vi "WPI_CameraSend Images To PC LoopCustom2.vi"(8 "error in (no error)":errorcluster, 11 "CameraDevRef":T1) -> ()   [LabVIEW 2015]
doc: "This VI is used to send images to the dashboard using the second enet port on the 8 slot controller. This is provided for compatibility, but is higher overhead than using the Camera MJPG approach.\n\nThis software is licensed. Open the labview\\readme\\WPI Robotics Library Open Source License.txt file for more information."
uses:
  <vilib>/Rock Robotics/WPI/Camera/WPI_CameraDevRef.ctl
  <vilib>/Rock Robotics/SystemInterfaces/NetworkCommunication/NetComm_UsageReport_ResourceType.ctl
  Robot Global Data.vi
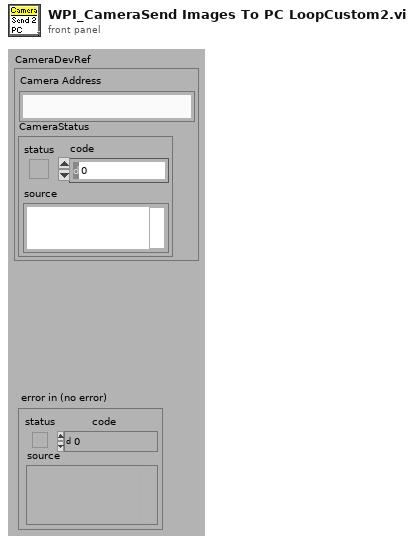
[diagram p1: front panel]
types:
  T1 = typedef "WPI_CameraDevRef.ctl" = cluster{"Camera Address":string, "CameraStatus":errorcluster}
  T2 = cluster{"fps":i32, "compression":i32, "compression 2":i32}
  T3 = typedef "NetComm_UsageReport_ResourceType.ctl" = enum8{"Controller", "Module", "Language", "CANPlugin", "Accelerometer", "ADXL345", "AnalogChannel", "AnalogTrigger", "AnalogTriggerOutput", "CANJaguar", "Compressor", "Counter", "Dashboard", "DigitalInput", "DigitalOutput", "DriverStationCIO", "DriverStationEIO", "DriverStationLCD", "Encoder", "GearTooth", "Gyro", "I2C", "Framework", "Jaguar", "Joystick", "Kinect", "KinectStick", "PIDController", "Preferences", "PWM", "Relay", "RobotDrive", "SerialPort", "Servo", "Solenoid", "SPI", "Task", "Ultrasonic", "Victor", "Button", "Command", "AxisCamera", "PCVideoServer", "SmartDashboard", "Talon", "HiTechnicColorSensor", "HiTechnicAccel", "HiTechnicCompass", "SRF08", "AnalogOutput", "Victor SP", "Talon SRX", "CAN Talon SRX", "ADXL362 Accel", "ADXRS450 Gyro", "Rev SPARK", "Mindsensors SD540", "Digital Filter"}
  T4 = enum16{"Update Mode", "Get Image", "Get Image Data"}
  T5 = typedef "Image Type" = u32
  T6 = typedef "IMAQ Image.ctl" = refnum<image>
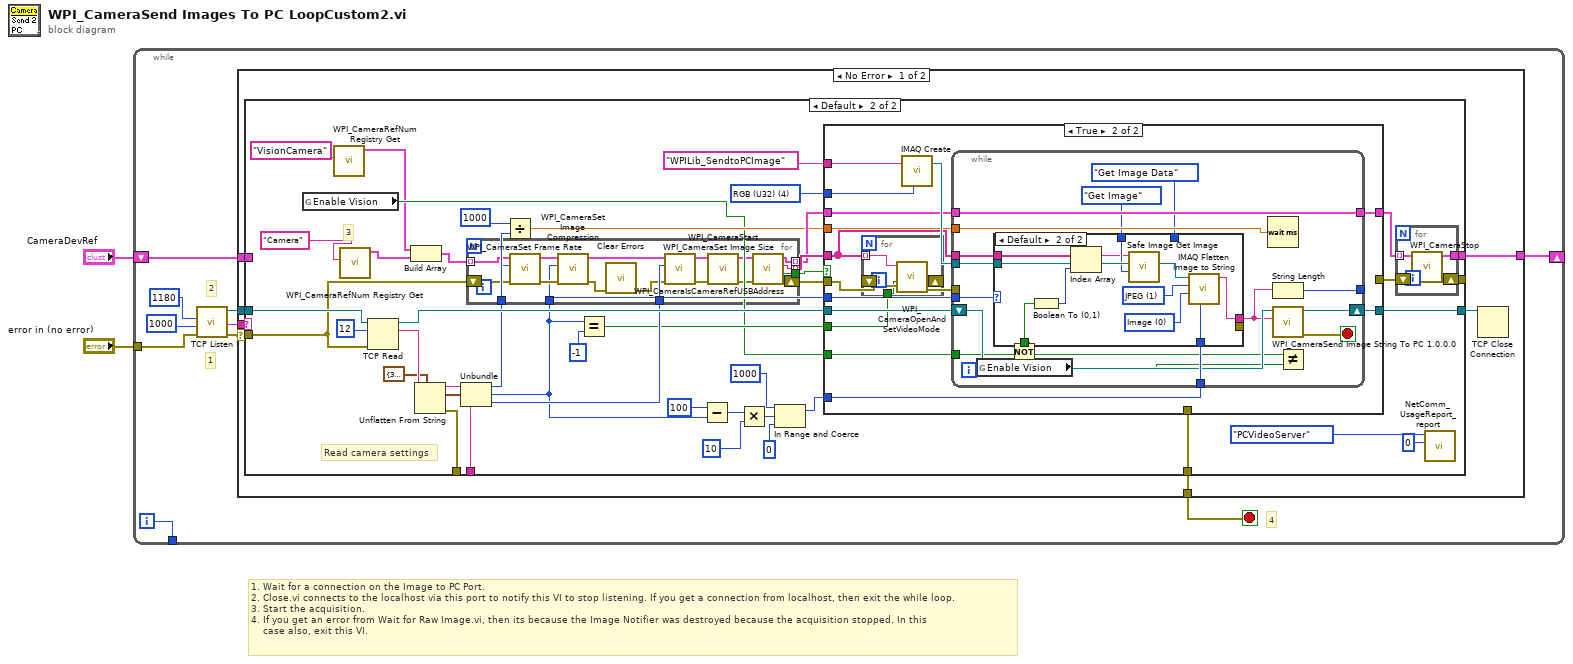
[diagram p0: block diagram]
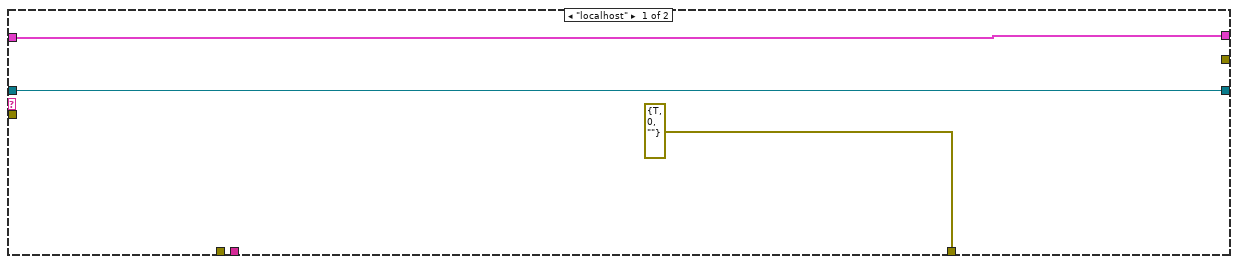
[diagram p2: hidden frame]
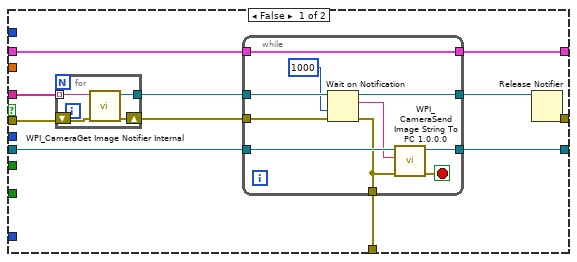
[diagram p3: hidden frame]
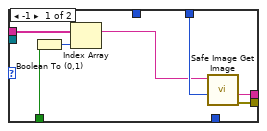
[diagram p4: hidden frame]
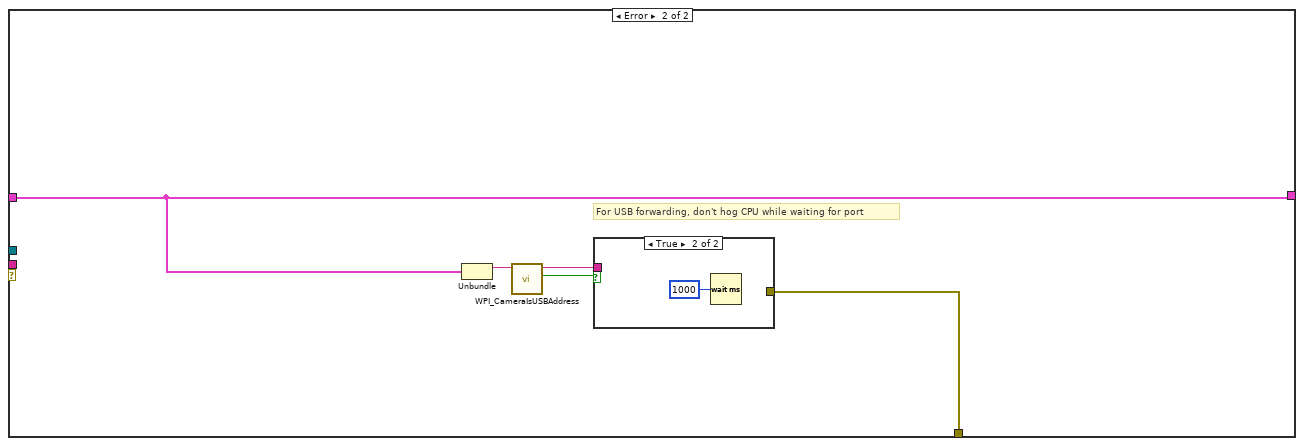
[diagram p5: hidden frame]
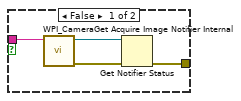
[diagram p6: hidden frame]
diagram:
  # "1. Wait for a connection on the Image to PC Port.\n2. Close.vi connects to the localhost via this port to notify this VI to stop listening. If you get a connection from localhost, then exit the while loop.\n3. Start the acquisition.\n4. If you get an error from Wait for Raw Image.vi, then its because the Image Notifier was destroyed because the acquisition stopped. In this\n    case also, exit this VI."
  n1 = while {
    tunnel: "error in (no error)" -> [w9]
    shift-right: [w12] -> _
    shift-left: "CameraDevRef" -> [w10]
    tunnel: [w3] -> _
    i -> [w3]
    stop <- w7 stop-if-true
    # "4"
    # "1"
    # "2"
    n2 = call <vilib>:"TCP Listen.vi"("error in (no error)"=w9, "timeout ms (wait forever: -1)"=u16 1000 ("port"), "port"=u16 1180) -> ("error out"=w5:errorcluster, "remote address"=w11:string, "connection ID"=w8:refnum<k5>)  [unwired: 1 in, 5 out]
    n3 = case shown="No Error" w5 {
      selector: w5 -> [w13 _]
      tunnel: [w19 w169] -> w12
      tunnel: w11 -> [w18 _]
      tunnel: w10 -> [w17 w169]
      tunnel: w8 -> [w16 _]
      tunnel: [w15 w170] -> w7
      frame No Error {
        n4 = case shown="Default" w18 {
          tunnel: [w22 w63] -> w19
          tunnel: w17 -> [w22 _]
          tunnel: w13 -> [_ w48]
          tunnel: w16 -> [w20 w52]
          tunnel: [errorcluster {"status"=TRUE, "code"=0, "source"=""} ("error out 2") w65] -> w15
          tunnel: [w20 w64] -> w14
          tunnel: [_ w62] -> _
          tunnel: [_ w31] -> _
          tunnel: [_ w30] -> _
          frame "localhost" {
          }
          frame Default {
            w57 = T5 4 items=["Grayscale (U8)", "Grayscale (I16)", "Grayscale (SGL)", "Complex (CSG)", "RGB (U32)", "HSL (U32)", "RGB (U64)", "Grayscale (U16)"] ("Image Type")
            # "Read camera settings"
            # "3"
            n5 = global read "Robot Global Data.vi" "Enable Vision"() -> (w29:bool)
            n6 = call <vilib>:"WPI_CameraRefNum Registry Get.vi"("refnum name"="VisionCamera") -> ("CameraDevRef"=w27:T1)  [unwired: 9 in, 1 out]
            n7 = call <vilib>:"WPI_CameraRefNum Registry Get.vi"("refnum name"="Camera") -> ("CameraDevRef"=w26:T1)  [unwired: 9 in, 1 out]
            n8 = TCP Read(connection ID=w52, bytes to read=12, error in (no error)=w48) -> (connection ID out=w51:refnum<k5>, data out=w49:string)  [unwired: 2 in, 1 out]
            n9 = Build Array(w27, w26) -> (w28:T1[])
            n10 = Unflatten From String(type=T2 {"fps"=30, "compression"=32, "compression 2"=32} ("Camera Settings"), binary string=w49) -> (rest of the binary string=w30:string, value=w47:T2, error out=w31:errorcluster)  [unwired: 3 in]
            n11 = Unbundle(w47) -> ("fps"=w44:i32, "compression"=w33:i32, "compression 2"=w46:i32)
            n12 = for {
              tunnel: [w87] -> w56 mode=indexing
              tunnel: [w86] -> w55
              tunnel: w46 -> [w76]
              tunnel: w44 -> [w75]
              tunnel: w33 -> [w74]
              shift-right: [w84] -> w54
              shift-left: w48 -> [w79]
              tunnel: w28 -> [w71] mode=indexing
              tunnel: [w70] -> w53 mode=indexing
              n13 = call <vilib>:"WPI_CameraSet Frame Rate.vi"("error in (no error)"=w79, "Frame Rate (fps)"=w75, "CameraDevRef"=w71) -> ("error out"=w78:errorcluster, "CameraDevRef Out"=w82:T1)  [unwired: 7 in]
              n14 = call <vilib>:"WPI_CameraSet Image Compression.vi"("error in (no error)"=w78, "Compression"=w74, "CameraDevRef"=w82) -> ("error out"=w73:errorcluster, "CameraDevRef Out"=w81:T1)  [unwired: 7 in]
              n15 = call <vilib>:"Clear Errors.vi"("error in (no error)"=w73) -> ("error out"=w72:errorcluster)  [unwired: 5 in, 1 out]
              n16 = call <vilib>:"WPI_CameraSet Image Size.vi"("error in (no error)"=w72, "Image Size"=w76, "CameraDevRef"=w81) -> ("error out"=w77:errorcluster, "CameraDevRef Out"=w80:T1)  [unwired: 7 in]
              n17 = call <vilib>:"WPI_CameraStart.vi"("error in (no error)"=w77, "CameraDevRef"=w80) -> ("error out"=w85:errorcluster, "CameraDevRef"=w83:T1)  [unwired: 8 out]
              n18 = call <vilib>:"WPI_CameraIsCameraRefUSBAddress.vi"("error in (no error)"=w85, "CameraDevRef"=w83) -> ("error out"=w84:errorcluster, "USB?"=w86:bool, "Camera Address Out"=w87:string, "CameraDevRef out"=w70:T1)  [unwired: 6 in]
            }
            n19 = Divide(x=u16 1000 ("port"), y=w44) -> (x/y=w43:dbl)
            n20 = Equal?(x=w33, y=-1) -> (x = y?=w32:bool)
            n21 = Subtract(x=100, y=w33) -> (x-y=w38:i32)
            n22 = Multiply(x=w38, y=10) -> (x*y=w40:i32)
            n23 = In Range and Coerce(upper limit=1000, x=w40, lower limit=0) -> (coerced(x)=w36:i32)  [unwired: 1 out]
            n24 = case shown="True" w55 {
              tunnel: w51 -> [w98 w127]
              tunnel: [w97 _] -> w65
              tunnel: [w96 w126] -> w64
              tunnel: w54 -> [w95 w117]
              tunnel: w56 -> [w93 w116]
              tunnel: [w92 w121] -> w25
              tunnel: w53 -> [w91 w122]
              tunnel: [w89 _] -> w61
              tunnel: "WPILib_SendtoPCImage" -> [_ w124]
              tunnel: w57 -> [_ w123]
              tunnel: w36 -> [_ w120]
              tunnel: w43 -> [_ w119]
              tunnel: w33 -> [_ w118]
              tunnel: w32 -> [_ w114]
              tunnel: w29 -> [_ w113]
              frame False {
                n25 = for {
                  tunnel: w93 -> [w100] mode=indexing
                  tunnel: [w99] -> w90
                  shift-right: [w101] -> w94
                  shift-left: w95 -> [w102]
                  n26 = call <vilib>:"WPI_CameraGet Image Notifier Internal.vi"("error in (no error)"=w102, "Camera Address"=w100) -> ("error out"=w101:errorcluster, "Image Notifier"=w99:refnum<notifier>)  [unwired: 8 out]
                }
                n27 = while {
                  tunnel: w94 -> [w108]
                  tunnel: w98 -> [w112]
                  tunnel: [w105] -> w97
                  tunnel: [w110] -> w96
                  tunnel: [w109] -> w92
                  tunnel: w91 -> [w109]
                  tunnel: w90 -> [w107]
                  tunnel: [w103] -> w88
                  stop <- w111 stop-if-true
                  n28 = Wait on Notification(notifier=w107, timeout in ms (-1)=1000 ("Timeout in ms (-1)"), error in (no error)=w108) -> (notifier out=w103:refnum<notifier>, notification=w106:string, error out=w105:errorcluster)  [unwired: 2 out]
                  n29 = call <vilib>:"WPI_CameraSend Image String To PC 1.0.0.0.vi"("error in (no error)"=w105, "String"=w106, "TCP Connection ID"=w112) -> ("error out"=w111:errorcluster, "TCP Connection ID out"=w110:refnum<k5>)  [unwired: 7 out]
                }
                n30 = Release Notifier(notifier=w88) -> (error out=w89:errorcluster)  [unwired: 1 in, 3 out]
              }
              frame True {
                n31 = for {
                  tunnel: w116 -> [w130] mode=indexing
                  tunnel: w114 -> [w128]
                  shift-right: [w129] -> w115
                  shift-left: w117 -> [w131]
                  n32 = call <vilib>:"WPI_CameraOpenAndSetVideoMode.vi"("error in (no error)"=w131, "USB JPEG"=w128, "Camera Address Out"=w130) -> ("error out"=w129:errorcluster)  [unwired: 8 in]
                }
                n33 = call "IMAQ Create"("Image Name"=w124, "Image Type"=w123) -> ("New Image"=w125:T6)  [unwired: 3 in, 1 out]
                n34 = while {
                  tunnel: w116 -> [w146]
                  shift-right: [w147] -> w126
                  shift-left: w127 -> [w141]
                  tunnel: w125 -> [w145]
                  tunnel: [w144] -> w121
                  tunnel: w122 -> [w144]
                  tunnel: w120 -> [w143]
                  tunnel: w119 -> [w142]
                  tunnel: [w139] -> _
                  tunnel: w118 -> [w138]
                  tunnel: w115 -> [_]
                  tunnel: w113 -> [w135]
                  stop <- w134 stop-if-true
                  n35 = global read "Robot Global Data.vi" "Enable Vision"() -> (w133:bool)
                  n36 = Not(x=w133) -> (.not. x?=w132:bool)
                  n37 = case shown="Default" w138 {
                    tunnel: [w153 w165] -> w140
                    tunnel: w146 -> [w154 w161]
                    tunnel: w145 -> [_ w160]
                    tunnel: w143 -> [_ w162]
                    tunnel: [w152 _] -> _
                    tunnel: T4."Get Image Data" ("Operation") -> [w151 _]
                    tunnel: T4."Get Image" ("Operation") -> [_ w158]
                    tunnel: w132 -> [w149 w156]
                    frame -1 {
                      n38 = Boolean To (0,1)(Boolean=w149) -> (0, 1=w148:i16)
                      n39 = Index Array(array=w154, index=w148) -> (element=w150:string)
                      n40 = call <vilib>:"Safe Image Get Image.vi"("Operation"=w151, "Session In"=w150) -> ("error out"=w152:errorcluster, "Image Data String"=w153:string)  [unwired: 6 in, 2 out]
                    }
                    frame Default {
                      w163 = 0 items=["Image", "Image and Vision Info", "Reference to Image"] ("Type of Flatten (Image and Vision Info)")
                      w164 = 1 items=["None", "JPEG", "PACKED BINARY"] ("Compression (None)")
                      n41 = Boolean To (0,1)(Boolean=w156) -> (0, 1=w155:i16)
                      n42 = Index Array(array=w161, index=w155) -> (element=w157:string)
                      n43 = call <vilib>:"Safe Image Get Image.vi"("Operation"=w158, "Image In"=w160, "Session In"=w157) -> ("Image Out"=w159:T6)  [unwired: 5 in, 3 out]
                      n44 = call "IMAQ Flatten Image to String"("Quality (750)"=w162, "Type of Flatten (Image and Vision Info)"=w163, "Compression (None)"=w164, "Image"=w159) -> ("Data String"=w165:string)  [unwired: 6 in, 1 out]
                    }
                  }
                  n45 = Wait (ms)(milliseconds to wait=w142) -> ()  [unwired: 1 out]
                  n46 = String Length(string=w140) -> (length=w139:i32)
                  n47 = call <vilib>:"WPI_CameraSend Image String To PC 1.0.0.0.vi"("String"=w140, "TCP Connection ID"=w141) -> ("error out"=w134:errorcluster, "TCP Connection ID out"=w147:refnum<k5>)  [unwired: 1 in, 7 out]
                  n48 = Not Equal?(x=w135, y=w133) -> ()  [unwired: 1 out]
                }
              }
            }
            n49 = for {
              tunnel: [w69] -> w63
              tunnel: w25 -> [w66] mode=indexing
              shift-right: [w68] -> w62
              shift-left: w61 -> [w67]
              n50 = call <vilib>:"WPI_CameraStop.vi"("error in (no error)"=w67, "CameraDevRef"=w66) -> ("error out"=w68:errorcluster, "CameraDevRef"=w69:T1)  [unwired: 8 out]
            }
            n51 = call <vilib>:"NetComm_UsageReport_report.vi"("Instance Number"=u8 0, "Resource Type"=NetComm_UsageReport_ResourceType."PCVideoServer") -> ()  [unwired: 10 in]
          }
        }
        n52 = TCP Close Connection(connection ID=w14) -> ()  [unwired: 1 in, 3 out]
      }
      frame Error {
        # "For USB forwarding, don't hog CPU while waiting for port"
        n53 = Unbundle(w169) -> ("Camera Address"=w168:string)  [unwired: 1 out]
        n54 = call <vilib>:"WPI_CameraIsUSBAddress.vi"("Camera Address In"=w168) -> ("USB?"=w166:bool, "Camera Address Out"=w167:string)  [unwired: 8 in, 1 out]
        n55 = case shown="True" w166 {
          tunnel: [w174 _] -> w170
          tunnel: w167 -> [w171 _]
          frame False {
            n56 = call <vilib>:"WPI_CameraGet Acquire Image Notifier Internal.vi"("Camera Address"=w171) -> ("error out"=w172:errorcluster, "Acquire Image Notifier"=w173:refnum<notifier>)  [unwired: 1 in, 8 out]
            n57 = Get Notifier Status(notifier=w173, error in (no error)=w172) -> (error out=w174:errorcluster)  [unwired: 4 out]
          }
          frame True {
            n58 = Wait (ms)(milliseconds to wait=u32 1000) -> ()  [unwired: 1 out]
          }
        }
      }
    }
  }
